vi "001_Calculate_DataSource.vi"(11 "Queue Ref In":T1={"UI"=refnum, "Message"=refnum, "Data"=refnum, "Caller"=refnum, "Name"="000 Common", "Data Path"=path "", "Class Path"=path "", "SubPanel"=refnum, "Project Name"="", "MNT"="", "Title"="", "Data Source"=refnum, "Queue List"={}, "VI"=refnum, "UE"=refnum}) -> ()   [LabVIEW 2020]
doc: "计算数据源"
uses:
  Alin/QMH/000 Module Data Type.ctl
  Alin/QMH/Queue Message.ctl
  <vilib>/Utility/miscctls.llb/LVRowAndColumnTypeDef.ctl
  <vilib>/Utility/file.llb/Read Delimited Spreadsheet (string).vi
  <vilib>/Utility/file.llb/Write Delimited Spreadsheet (string).vi
panel:
  in  "Formular List Refresh":bool
  in  "Formular Group Delete":bool
  in  "Formular Group Add":bool
  in  "Formular List":i32(listbox)
  in  "Warning Edit":bool
  in  "Formular Delete":bool
  in  "Formular Export":bool
  in  "Formular Import":bool
  in  "Formular Add":bool
  in  "Formular":i32(listbox)
  in  "Search":bool
  in  "Search Info":string
  in  "All Formular":i32(listbox)
  out "Delay":i32 format="Delay：%.0f ms"
  out "Numbers":i32 format="Sum：%.0f"
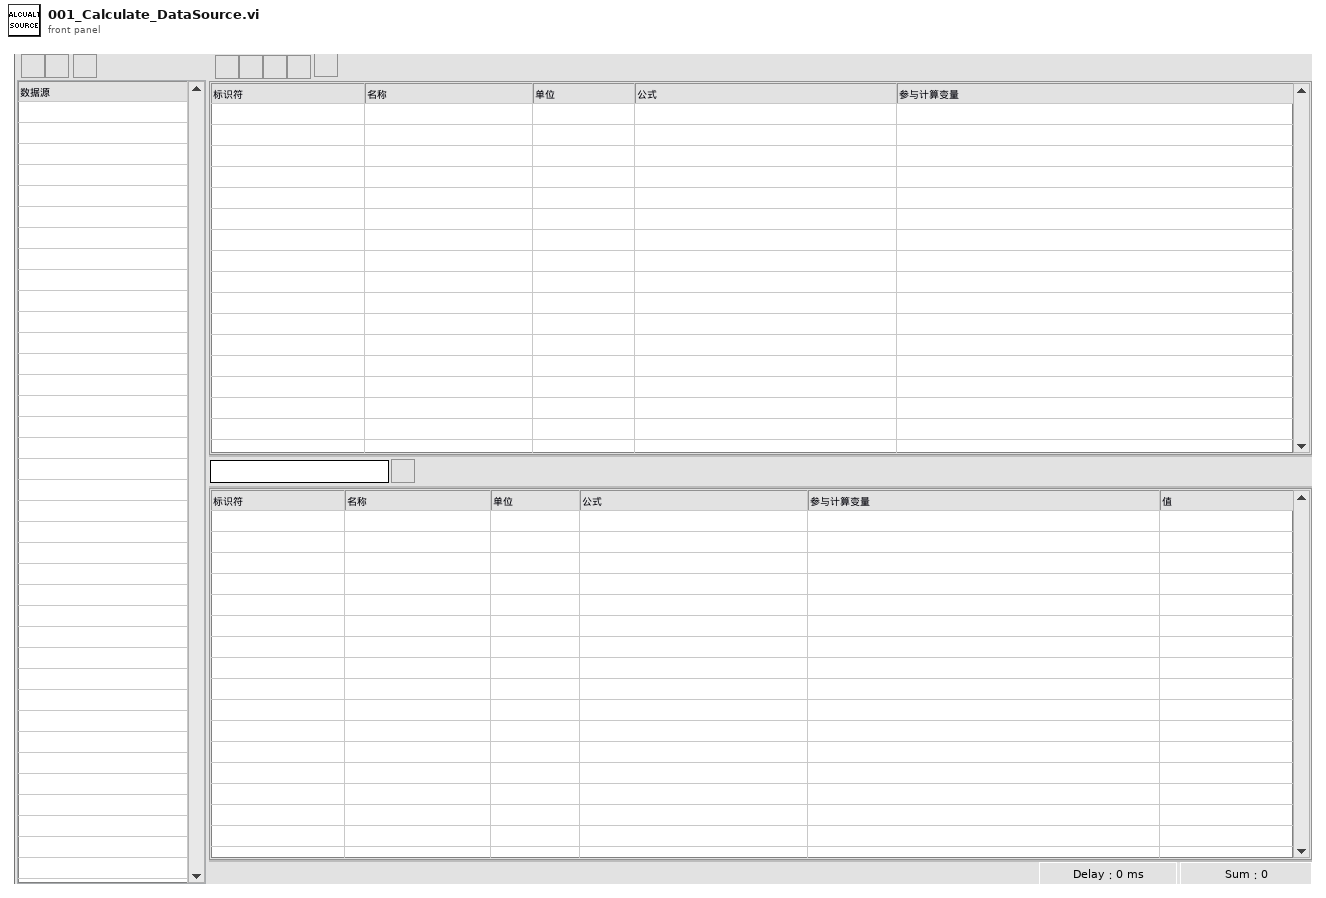
[diagram p1: front panel]
types:
  T1 = typedef "000 Module Data Type.ctl" = cluster{"UI":refnum<queue>, "Message":refnum<queue>, "Data":refnum<queue>, "Caller":refnum<queue>, "Name":string, "Data Path":path, "Class Path":path, "SubPanel":refnum<vi>, "Project Name":string, "MNT":string, "Title":string, "Data Source":refnum<queue>, "Queue List":map{string, refnum<queue>}, "VI":refnum<vi>, "UE":refnum<user-event>}
  T2 = cluster{"Queue":T1, "Formular":string[][], "Formular List":string[], "Last Time":u32, "Delay":u32, "Data Refresh":string}
  T3 = typedef "eventvkey.ctl" = enum16{"ASCII", "Enter", "Return", "Shift", "Ctrl", "Alt", "Cmd", "Opt", "Caps", "NumLock", "Clear", "Break", "Up", "Down", "Left", "Right", "Insert", "Delete", "Home", "End", "PageUp", "PageDown", "Escape", "Help", "Pause", "ScrollLock", "F1", "F2", "F3", "F4", "F5", "F6", "F7", "F8", "F9", "F10", "F11", "F12", "F13", "F14", "F15", "F16", "F17", "F18", "F19", "F20", "F21", "F22", "F23", "F24", "Play", "VolumeUp", "VolumeDown", "Mute", "Two Byte Char"}
  T4 = cluster{"Shift":bool, "Ctrl":bool, "Alt":bool, "Cmd":bool, "Opt":bool}
  T5 = typedef "LVPoint32TypeDef.ctl" = cluster{"Horizontal":i32, "Vertical":i32}
  T6 = typedef "LVRowAndColumnTypeDef.ctl" = cluster{"Row":i32, "Column":i32}
  T7 = cluster{"Formular":string[][], "Queue":T1, "FormularRef":refnum<vi>, "Formular ListRef":refnum<vi>, "Formular List":string[], "ForList Value":i32}
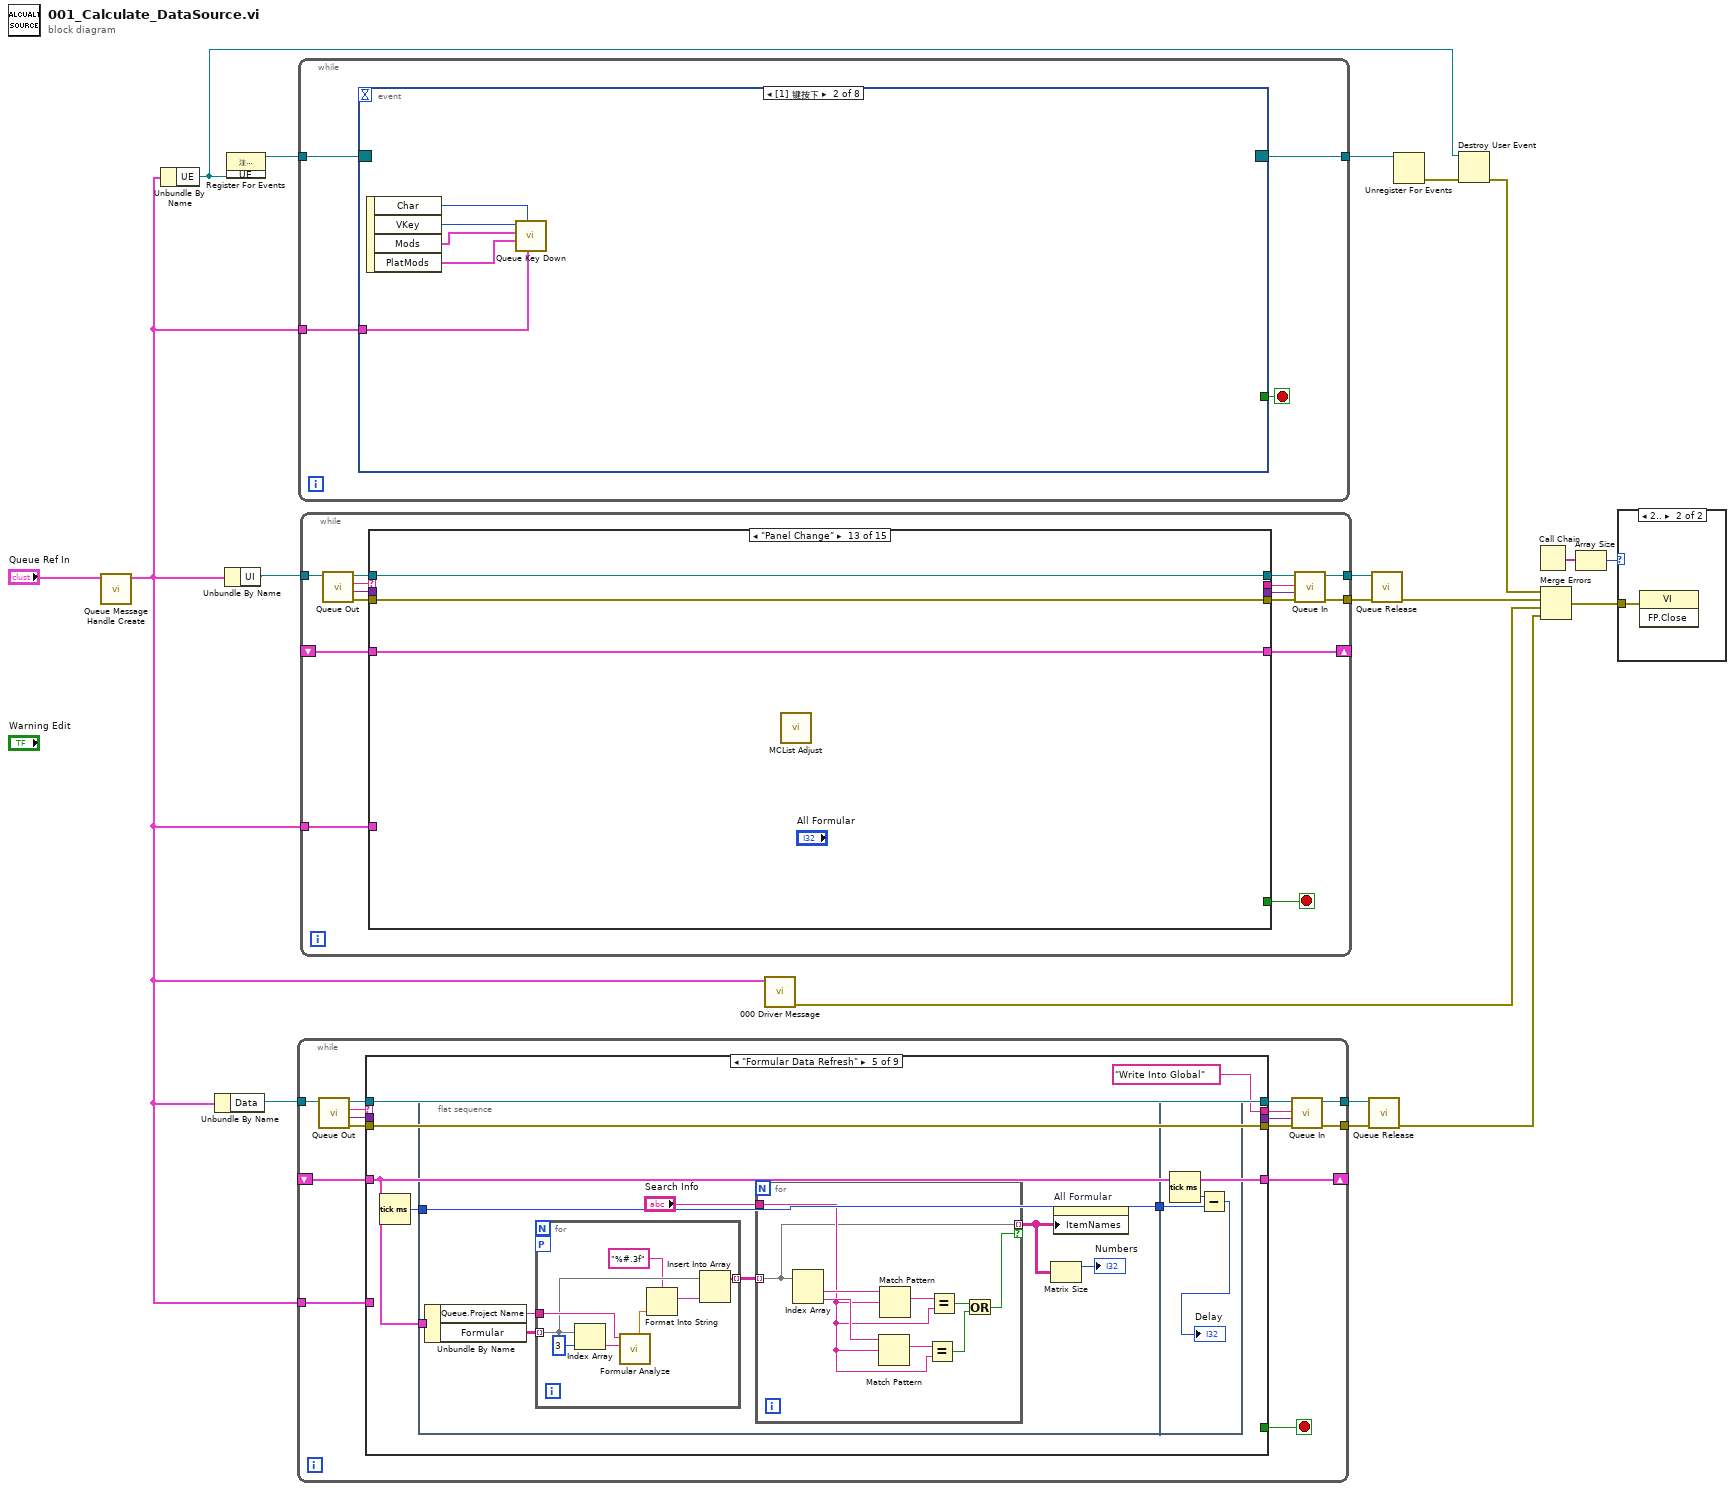
[diagram p0: block diagram]
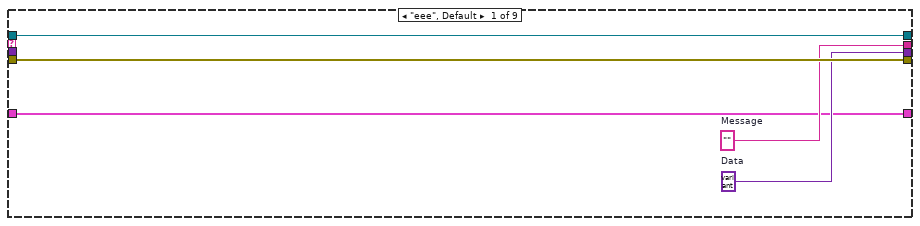
[diagram p2: hidden frame]
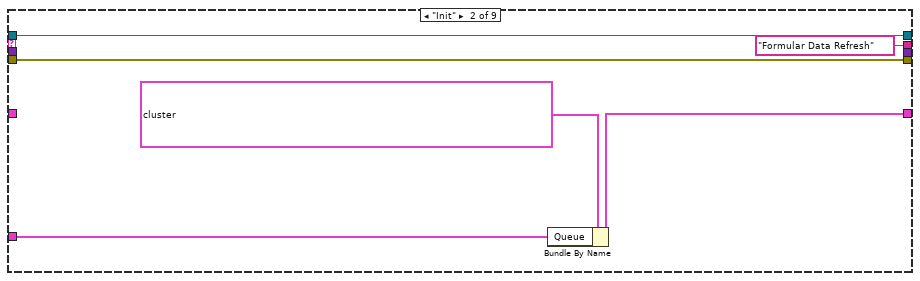
[diagram p3: hidden frame]
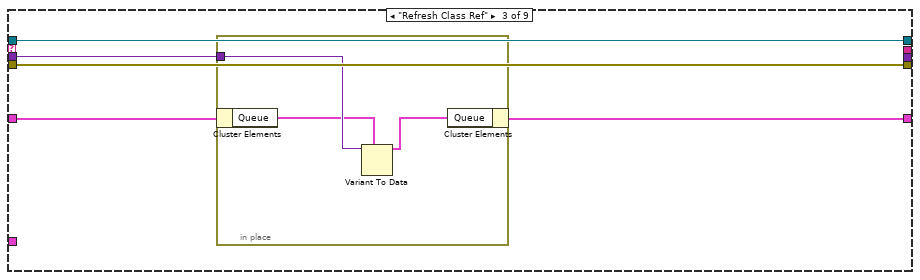
[diagram p4: hidden frame]
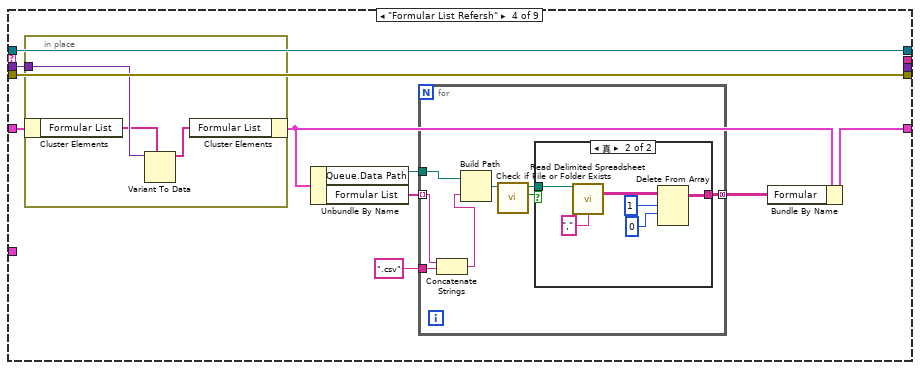
[diagram p5: hidden frame]
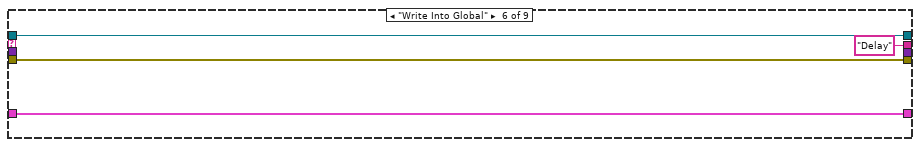
[diagram p7: hidden frame]
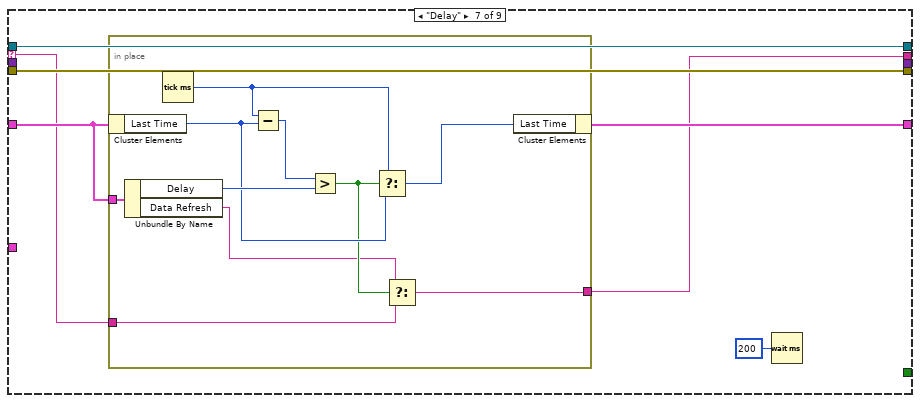
[diagram p8: hidden frame]
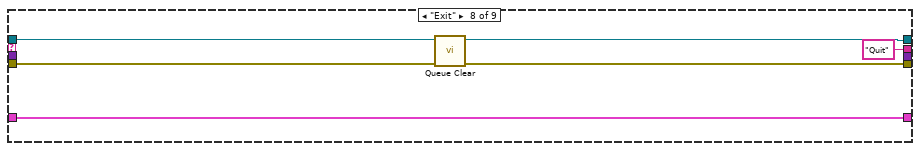
[diagram p9: hidden frame]
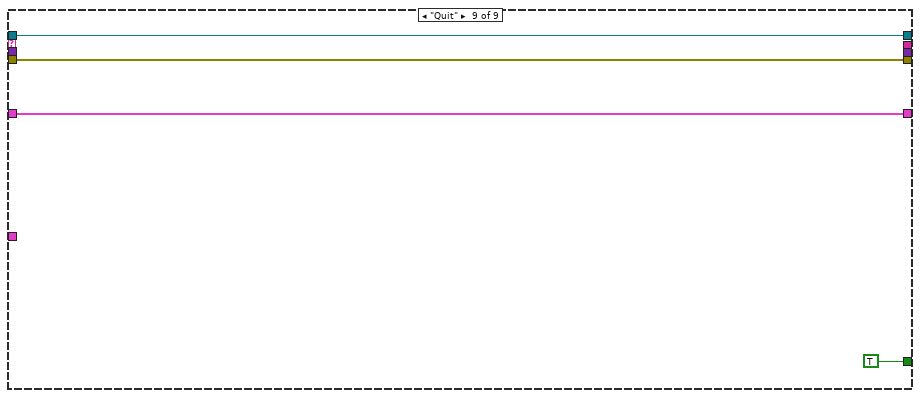
[diagram p10: hidden frame]
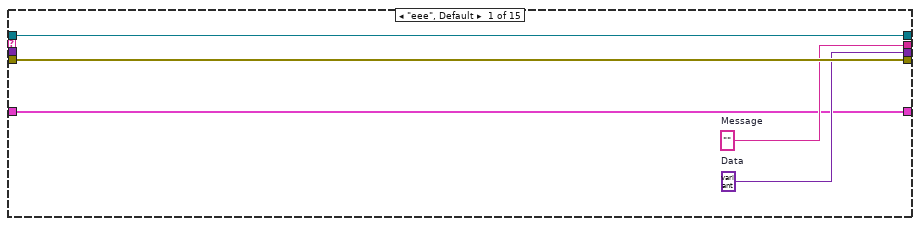
[diagram p12: hidden frame]
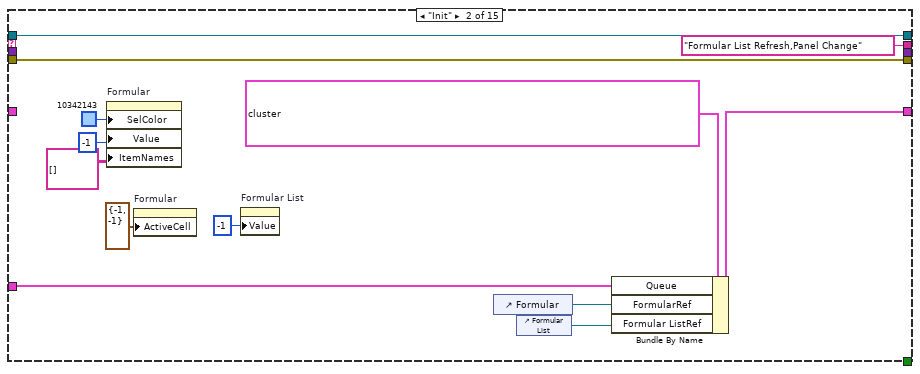
[diagram p13: hidden frame]
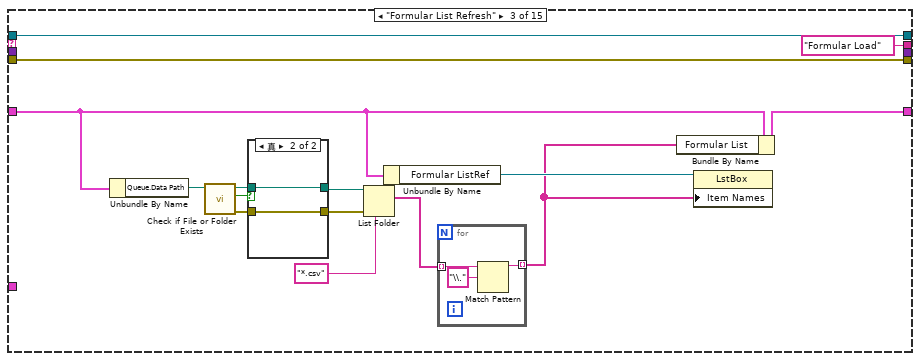
[diagram p14: hidden frame]
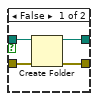
[diagram p15: hidden frame]
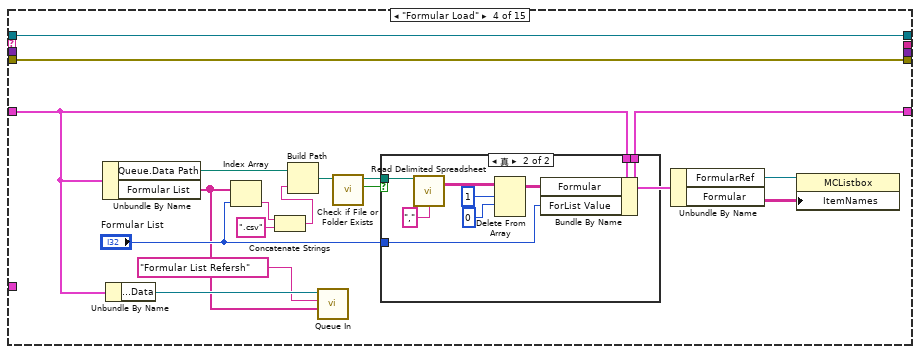
[diagram p16: hidden frame]
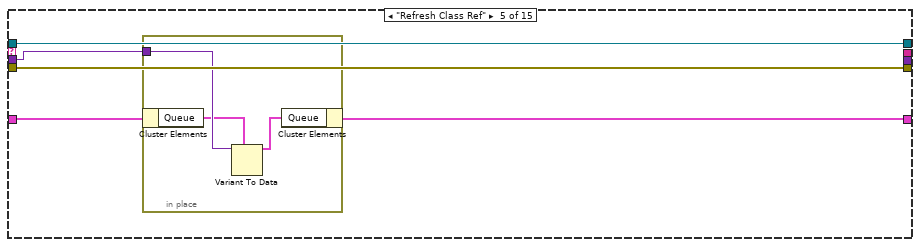
[diagram p18: hidden frame]
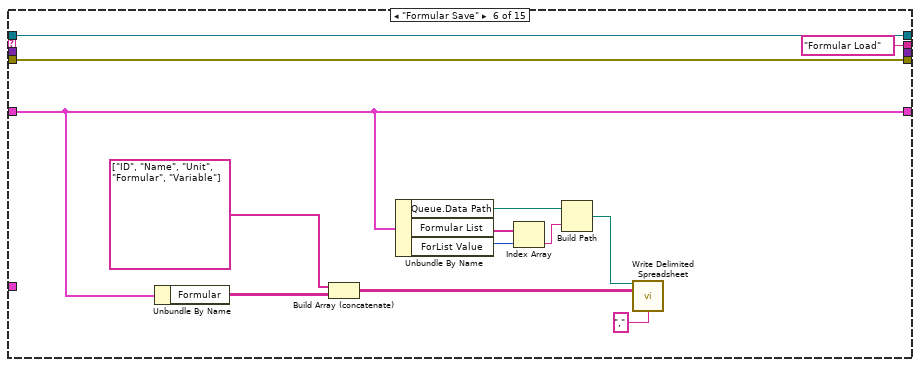
[diagram p19: hidden frame]
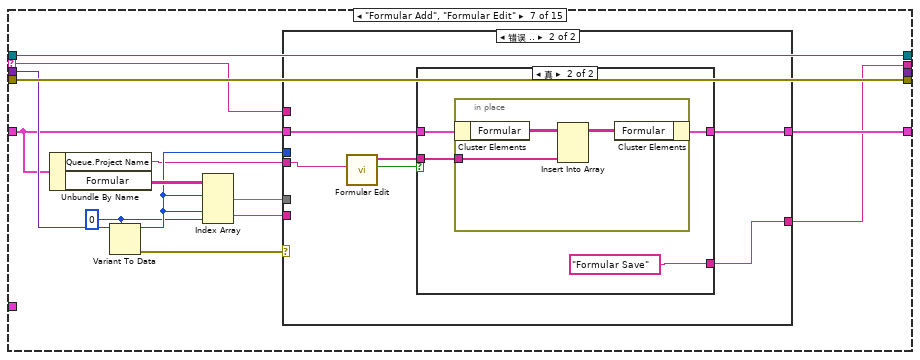
[diagram p20: hidden frame]
diagram:
  n1 = call "Queue Message Handle Create.vi"("Queue Ref In"="Queue Ref In") -> ("Queue Ref Out"=w1:T1)  [unwired: 9 in, 1 out]
  n2 = Unbundle By Name(w1) -> ("UE"=w2:refnum<user-event>)
  n3 = Unbundle By Name(w1) -> ("Data"=w17:refnum<queue>)
  n4 = Unbundle By Name(w1) -> ("UI"=w9:refnum<queue>)
  n5 = register-events(w2) -> (reference out=w4:refnum<event-registration>)  [unwired: 2 in, 1 out]
  n6 = while {
    tunnel: w17 -> [w30]
    tunnel: [w27] -> w15
    tunnel: [w26] -> w16
    shift-right: [w22] -> _
    shift-left: _ -> [w21]
    tunnel: w1 -> [w20]
    stop <- w34 stop-if-true
    n7 = call "Queue Out.vi"("Queue In"=w30) -> ("error out"=w33:errorcluster, "Data"=w31:variant, "Message"=w32:string, "Queue Out"=w29:refnum<queue>)  [unwired: 6 in, 1 out]
    n8 = case shown="\"Formular Data Refresh\"" w32 {
      selector: w32 -> [_ _ _ _ _ _ w120 _ _]
      tunnel: w29 -> [w39 w45 w50 w63 w86 w118 w125 w140 w144]
      tunnel: w33 -> [w38 w44 w49 w62 w85 w117 w124 w138 w145]
      tunnel: [w39 w45 w50 w63 w86 w118 w125 w139 w144] -> w28
      tunnel: [w38 w44 w49 w62 w85 w117 w124 w137 w145] -> w25
      tunnel: [w37 "Formular Data Refresh" ("Message") _ _ "Write Into Global" ("Message") "Delay" ("Data Refresh") w119 "Quit" _] -> w24
      tunnel: [_ _ _ _ _ _ _ _ TRUE] -> w34
      tunnel: [w36 _ _ _ _ _ _ _ _] -> w23
      tunnel: w31 -> [_ _ w46 w60 _ _ _ _ _]
      tunnel: [w35 w42 w47 w56 w83 w116 w122 w136 w142] -> w22
      tunnel: w21 -> [w35 _ w48 w61 w83 w116 w121 w136 w142]
      tunnel: w20 -> [_ w41 _ _ _ _ _ _ _]
      frame "eee", Default {
        w36 = variant  # Data
        w37 = ""  # Message
      }
      frame "Init" {
        n9 = Bundle By Name(cluster=T2 {"Queue"={"UI"=refnum, "Message"=refnum, "Data"=refnum, "Caller"=refnum, "Name"="000 Common", "Data Path"=path "", "Class Path"=path "", "SubPanel"=refnum, "Project Name"="", "MNT"="", "Title"="", "Data Source"=refnum, "Queue List"={}, "VI"=refnum, "UE"=refnum}, "Formular"=[], "Formular List"=[], "Last Time"=0, "Delay"=500, "Data Refresh"="Formular Data Refresh"}, "Queue"=w41) -> (w42:T2)
      }
      frame "Refresh Class Ref" {
        n10 = in-place {
          in-place-border: w46 -> [w53]
          n11 = in-place-cluster #1(w48) -> ("Queue"=w52:T1)
          n12 = Variant To Data(type=w52, Variant=w53) -> (data=w51:T1)  [unwired: 1 in, 1 out]
          n13 = in-place-cluster #1("Queue"=w51) -> (w47:T2)
        }
      }
      frame "Formular List Refersh" {
        n14 = in-place {
          in-place-border: w60 -> [w80]
          n15 = in-place-cluster #2(w61) -> ("Formular List"=w79:string[])
          n16 = Variant To Data(type=w79, Variant=w80) -> (data=w78:string[])  [unwired: 1 in, 1 out]
          n17 = in-place-cluster #2("Formular List"=w78) -> (w59:T2)
        }
        n18 = Unbundle By Name(w59) -> ("Queue.Data Path"=w58:path, "Formular List"=w57:string[])
        n19 = for {
          tunnel: w58 -> [w70]
          tunnel: w57 -> [w65] mode=indexing
          tunnel: [w67] -> w55 mode=concatenating
          tunnel: ".csv" ("字符串") -> [w66]
          n20 = Concatenate Strings(w65, w66) -> (w64:string)
          n21 = Build Path(base path=w70, name or relative path=w64) -> (appended path=w71:path)
          n22 = call <vilib>:"Check if File or Folder Exists.vi"("path"=w71) -> ("file or folder exists?"=w69:bool, "dup path"=w68:path)  [unwired: 8 in, 1 out]
          n23 = case shown="真" w69 {
            tunnel: w68 -> [_ w74]
            tunnel: [_ w72] -> w67
            frame False {
            }
            frame True {
              n24 = call-poly <vilib>:"Read Delimited Spreadsheet.vi"("file path (dialog if empty)"=w74, "delimiter (\\t)"="," ("delimiter (\\t)")) -> ("all rows"=w73:string[][])  [unwired: 8 in, 5 out]
              n25 = Delete From Array(array=w73, length=1 ("长度"), index (row)=0 ("索引 (行)")) -> (array with subset deleted=w72:string[][])  [unwired: 1 in, 1 out]
            }
          }
        }
        n26 = Bundle By Name(cluster=w59, "Formular"=w55) -> (w56:T2)
      }
      frame "Formular Data Refresh" {
        n27 = Tick Count (ms)() -> (millisecond timer value=w82:u32)
        n28 = flat-sequence {
          tunnel: w83 -> [w94]
          tunnel: w82 -> [w87]
          tunnel: [w87] -> w81
          tunnel: w81 -> [w113]
          frame #0 {
            n29 = Unbundle By Name(w94) -> ("Queue.Project Name"=w92:string, "Formular"=w93:string[][])
            n30 = for {
              workers-P: _ -> [_]
              tunnel: w93 -> [w108] mode=indexing
              tunnel: w92 -> [w109]
              tunnel: [w107] -> w91 mode=indexing
              n31 = Index Array(array=w108, index=3 ("索引")) -> (element=w110:string)
              n32 = call "Formular Analyze.vi"("Formular"=w110, "Project"=w109) -> ("Value"=w105:dbl)  [unwired: 5 in, 4 out]
              n33 = Format Into String(format string="%#.3f" ("格式字符串"), w105) -> (resulting string=w104:string)  [unwired: 2 in, 1 out]
              n34 = Insert Into Array(array=w108, new element=w104) -> (w107:string[])  [unwired: 1 in]
            }
            n35 = for {
              tunnel: w91 -> [w97] mode=indexing
              tunnel: "Search Info" -> [w100]
              tunnel: [w97] -> w89 mode=indexing if=w96
              n36 = Index Array(array=w97) -> (element #1=w103:string, element #2=w102:string)  [unwired: 2 in]
              n37 = Match Pattern(string=w102, regular expression=w100) -> (match substring=w95:string)  [unwired: 1 in, 3 out]
              n38 = Match Pattern(string=w103, regular expression=w100) -> (match substring=w101:string)  [unwired: 1 in, 3 out]
              n39 = Equal?(x=w95, y=w100) -> (x = y?=w98:bool)
              n40 = Equal?(x=w101, y=w100) -> (x = y?=w99:bool)
              n41 = Or(x=w99, y=w98) -> (x .or. y?=w96:bool)
            }
            n42 = Matrix Size(0:w89) -> (1:→"Numbers":i32)  [unwired: 1 out]
            n43 = property on="All Formular" class="MCListbox (严格)"("ItemNames"=w89) -> ()  [unwired: 2 in, 2 out]
          }
          frame #1 {
            n44 = Tick Count (ms)() -> (millisecond timer value=w114:u32)
            n45 = Subtract(x=w114, y=w113) -> (x-y=→"Delay":u32)
          }
        }
      }
      frame "Write Into Global" {
      }
      frame "Delay" {
        n46 = in-place {
          in-place-border: w121 -> [w134]
          in-place-border: w120 -> [w128]
          in-place-border: [w127] -> w119
          n47 = in-place-cluster #3(w121) -> ("Last Time"=w130:u32)
          n48 = Unbundle By Name(w134) -> ("Delay"=w133:u32, "Data Refresh"=w126:string)
          n49 = Tick Count (ms)() -> (millisecond timer value=w132:u32)
          n50 = Subtract(x=w132, y=w130) -> (x-y=w135:u32)
          n51 = Greater?(x=w135, y=w133) -> (0:w129:bool)
          n52 = Select(t=w132, s=w129, f=w130) -> (s? t:f=w131:u32)
          n53 = Select(t=w126, s=w129, f=w128) -> (s? t:f=w127:string)
          n54 = in-place-cluster #3("Last Time"=w131) -> (w122:T2)
        }
        n55 = Wait (ms)(milliseconds to wait=u32 200 ("等待时间（毫秒）")) -> ()  [unwired: 1 out]
      }
      frame "Exit" {
        n56 = call "Queue Clear.vi"("error in (no error)"=w138, "Queue In"=w140) -> ("error out"=w137:errorcluster, "Queue Out"=w139:refnum<queue>)  [unwired: 8 in]
      }
      frame "Quit" {
      }
    }
    n57 = call "Queue In.vi"("error in (no error)"=w25, "Data"=w23, "Message"=w24, "Queue In"=w28) -> ("error out"=w26:errorcluster, "Queue Out"=w27:refnum<queue>)  [unwired: 6 in]
  }
  n58 = while {
    tunnel: w4 -> [w149]
    tunnel: [w147] -> w5
    tunnel: w1 -> [w146]
    stop <- w148 stop-if-true
    n59 = event shown="[1] 键按下" {
      selector: w149 -> [_ _ _ _ _ _ _ _]
      dyn-events: [_ _ _ _ _ _ _ _] -> w147
      timeout: _ -> [_ _ _ _ _ _ _ _]
      tunnel: [_ _ _ w158 _ _ _ _] -> w148
      tunnel: w146 -> [_ w150 w157 _ w163 w179 w185 w189]
      event Timeout {
        n60 = event-data() -> ()  [unwired: 1 in, 1 out]
      }
      event Key Down {
        n61 = event-data() -> ("Char"=w154:i16, "VKey"=w153:T3, "Mods"=w152:cluster{"Num Pad":bool, "Menu Key":bool}, "PlatMods"=w151:T4)  [unwired: 1 in]
        n62 = call "Queue Key Down.vi"("Queue Ref Out"=w150, "C"=w154, "Platform Key"=w151, "Group Key"=w152, "V Key"=w153) -> ()  [unwired: 6 in, 1 out]
      }
      event Panel Resize {
        n63 = event-data() -> ()  [unwired: 1 in, 1 out]
        n64 = Unbundle By Name(w157) -> ("Message"=w156:refnum<queue>)
        n65 = call "Queue In.vi"("Message"="Panel Change", "Queue In"=w156) -> ()  [unwired: 8 in, 2 out]
      }
      event User Event {
        n66 = event-data() -> ("Message"=w160:string)  [unwired: 1 in]
        n67 = Equal?(x=w160, y="Exit") -> (x = y?=w158:bool)
      }
      event Panel Close? {
        n68 = event-data() -> ()  [unwired: 1 in, 1 out]
        n69 = Call Chain() -> (call chain=w165:string[])
        n70 = Array Size(array=w165) -> (size(s)=w164:i32)
        n71 = case shown="1" w164 {
          tunnel: w163 -> [w169 w172]
          tunnel: [w168 w171] -> w162
          tunnel: ["Panel Hidden" ("Message") "Exit Prepare" ("Message")] -> w161
          frame 2, Default {
            n72 = Unbundle By Name(w169) -> ("Message"=w168:refnum<queue>)
          }
          frame 1 {
            n73 = Unbundle By Name(w172) -> ("Message"=w171:refnum<queue>)
          }
        }
        n74 = call "Queue In.vi"("Message"=w161, "Queue In"=w162) -> ()  [unwired: 8 in, 2 out]
        n75 = event-data("Discard?"=TRUE ("放弃？")) -> ()  [unwired: 1 in, 1 out]
      }
      event "Formular": Double Click {
        n76 = event-data() -> ("CtlRef"=w177:refnum<vi>, "Coords"=w176:T5)  [unwired: 1 in]
        n77 = Unbundle By Name(w179) -> ("UI"=w178:refnum<queue>)
        n78 = invoke class="MCListbox (严格)" method="Point To Row Column"(reference=w177, "Point"=w176) -> ("CellPosition"=w175:T6)  [unwired: 5 in, 6 out]
        n79 = Unbundle By Name(w175) -> ("Column"=w174:i32, "Row"=w173:i32)
        n80 = case shown="3" w174 {
          tunnel: w178 -> [_ w182]
          tunnel: w173 -> [_ w180]
          frame 0, Default {
          }
          frame 3 {
            n81 = call "Queue In.vi"("Data"=w180, "Message"="Formular Edit", "Queue In"=w182) -> ()  [unwired: 7 in, 2 out]
          }
        }
      }
      event "Formular Add", "Formular Group Add", "Formular Group Delete", "Formular Import", "Formular Export", "Formular Delete", "Formular List Refresh": Value Change {
        n82 = event-data() -> ("CtlRef"=w186:refnum<vi>)  [unwired: 1 in]
        n83 = property class="Bool"(reference=w186) -> ("Label.Text"=w183:string)  [unwired: 1 in, 2 out]
        n84 = Unbundle By Name(w185) -> ("UI"=w184:refnum<queue>)
        n85 = call "Queue In.vi"("Message"=w183, "Queue In"=w184) -> ()  [unwired: 8 in, 2 out]
      }
      event "Formular List": Value Change {
        n86 = event-data() -> ()  [unwired: 1 in, 1 out]
        n87 = Unbundle By Name(w189) -> ("UI"=w188:refnum<queue>)
        n88 = call "Queue In.vi"("Message"="Formular Load", "Queue In"=w188) -> ()  [unwired: 8 in, 2 out]
      }
    }
  }
  n89 = while {
    tunnel: w9 -> [w200]
    tunnel: [w197] -> w7
    tunnel: [w196] -> w8
    tunnel: w1 -> [w192]
    shift-right: [w191] -> _
    shift-left: _ -> [w190]
    stop <- w204 stop-if-true
    n90 = call "Queue Out.vi"("Queue In"=w200) -> ("error out"=w203:errorcluster, "Data"=w201:variant, "Message"=w202:string, "Queue Out"=w199:refnum<queue>)  [unwired: 6 in, 1 out]
    n91 = case shown="\"Panel Change\"" w202 {
      selector: w202 -> [_ _ _ _ _ _ w298 _ _ _ _ _ _ w451 _]
      tunnel: w199 -> [w209 w222 w237 w263 w278 w294 w308 w359 w381 w391 w413 w437 w448 w458 w464]
      tunnel: w203 -> [w208 w221 w236 w262 w277 w293 w307 w358 w380 w390 w412 w436 w447 w456 w465]
      tunnel: [w209 w222 w237 w263 w278 w294 w308 w359 w381 w391 w413 w437 w448 w457 w464] -> w198
      tunnel: [w208 w221 w236 w262 w277 w293 w307 w358 w380 w390 w412 w436 w447 w455 w465] -> w195
      tunnel: [w207 "Formular List Refresh,Panel Change" ("Message") "Formular Load" ("Message") _ _ "Formular Load" ("Message") w301 "Formular List Refresh" ("Message") "Formular List Refresh" ("Message") _ w404 w433 _ "Quit" _] -> w194
      tunnel: [_ _ _ _ _ _ _ _ _ _ _ _ _ _ TRUE] -> w204
      tunnel: [w206 _ _ _ _ _ _ _ _ _ _ _ _ _ _] -> w193
      tunnel: w201 -> [_ _ _ _ w274 _ w306 _ _ _ _ _ _ _ _]
      tunnel: w192 -> [_ w210 _ _ _ _ _ _ _ _ _ _ _ _ _]
      tunnel: [w205 w218 w226 w258 w275 w290 w302 w355 w379 w384 w406 w435 w446 w449 w462] -> w191
      tunnel: w190 -> [w205 _ w229 w253 w276 w290 w305 w355 w379 w385 w407 w434 w446 w449 w462]
      frame "eee", Default {
        w206 = variant  # Data
        w207 = ""  # Message
      }
      frame "Init" {
        n92 = property on="Formular" class="MCListbox (严格)"("SelColor"=u32 10342143 ("选择颜色"), "Value"=-1 ("Formular"), "ItemNames"=string[][] [] ("项名")) -> ()  [unwired: 2 in, 2 out]
        n93 = property on="Formular" class="MCListbox (严格)"("ActiveCell"=T6 {"Row"=-1, "Column"=-1} ("活动单元格:活动单元格")) -> ()  [unwired: 2 in, 2 out]
        n94 = property on="Formular List" class="LstBox (严格)"("Value"=-1 ("Formular List")) -> ()  [unwired: 2 in, 2 out]
        n95 = control-ref of="Formular"() -> (w216:refnum<vi>)
        n96 = control-ref of="Formular List"() -> (w215:refnum<vi>)
        n97 = Bundle By Name(cluster=T7 {"Formular"=[], "Queue"={"UI"=refnum, "Message"=refnum, "Data"=refnum, "Caller"=refnum, "Name"="000 Common", "Data Path"=path "", "Class Path"=path "", "SubPanel"=refnum, "Project Name"="", "MNT"="", "Title"="", "Data Source"=refnum, "Queue List"={}, "VI"=refnum, "UE"=refnum}, "FormularRef"=refnum, "Formular ListRef"=refnum, "Formular List"=[], "ForList Value"=0}, "Queue"=w210, "FormularRef"=w216, "Formular ListRef"=w215) -> (w218:T7)
      }
      frame "Formular List Refresh" {
        n98 = Unbundle By Name(w229) -> ("Queue.Data Path"=w235:path)
        n99 = call <vilib>:"Check if File or Folder Exists.vi"("path"=w235) -> ("error out"=w232:errorcluster, "file or folder exists?"=w234:bool, "dup path"=w233:path)  [unwired: 8 in]
        n100 = case shown="真" w234 {
          tunnel: w233 -> [w244 w246]
          tunnel: w232 -> [w243 w245]
          tunnel: [w241 w246] -> w231
          tunnel: [w242 w245] -> w230
          frame False {
            n101 = Create Folder(path (use dialog)=w244, error in=w243) -> (created path=w241:path, error out=w242:errorcluster)  [unwired: 1 in, 1 out]
          }
          frame True {
          }
        }
        n102 = List Folder(path=w231, pattern="*.csv" ("类型"), error in=w230) -> (filenames=w224:string[])  [unwired: 1 in, 3 out]
        n103 = Unbundle By Name(w229) -> ("Formular ListRef"=w228:refnum<vi>)
        n104 = for {
          tunnel: w224 -> [w240] mode=indexing
          tunnel: [w238] -> w223 mode=indexing
          n105 = Match Pattern(string=w240, regular expression="\\." ("正则表达式")) -> (before substring=w238:string)  [unwired: 1 in, 3 out]
        }
        n106 = Bundle By Name(cluster=w229, "Formular List"=w223) -> (w226:T7)
        n107 = property class="LstBox"(reference=w228, "Item Names"=w223) -> ()  [unwired: 1 in, 2 out]
      }
      frame "Formular Load" {
        n108 = Unbundle By Name(w253) -> ("Queue.Data Path"=w261:path, "Formular List"=w251:string[])
        n109 = Unbundle By Name(w253) -> ("Queue.Data"=w252:refnum<queue>)
        n110 = Index Array(array=w251, index="Formular List") -> (element=w249:string)
        n111 = Concatenate Strings(w249, ".csv" ("字符串")) -> (w247:string)
        n112 = Build Path(base path=w261, name or relative path=w247) -> (appended path=w256:path)
        n113 = call "Queue In.vi"("Data"=w251, "Message"="Formular List Refersh", "Queue In"=w252) -> ()  [unwired: 7 in, 2 out]
        n114 = call <vilib>:"Check if File or Folder Exists.vi"("path"=w256) -> ("file or folder exists?"=w255:bool, "dup path"=w254:path)  [unwired: 8 in, 1 out]
        n115 = case shown="真" w255 {
          tunnel: w253 -> [w264 w273]
          tunnel: [w264 w267] -> w258
          tunnel: "Formular List" -> [_ w266]
          tunnel: w254 -> [_ w265]
          frame False {
          }
          frame True {
            n116 = call-poly <vilib>:"Read Delimited Spreadsheet.vi"("file path (dialog if empty)"=w265, "delimiter (\\t)"="," ("delimiter (\\t)")) -> ("all rows"=w268:string[][])  [unwired: 8 in, 5 out]
            n117 = Delete From Array(array=w268, length=1 ("长度"), index (row)=0 ("索引 (行)")) -> (array with subset deleted=w271:string[][])  [unwired: 1 in, 1 out]
            n118 = Bundle By Name(cluster=w273, "Formular"=w271, "ForList Value"=w266) -> (w267:T7)
          }
        }
        n119 = Unbundle By Name(w258) -> ("FormularRef"=w259:refnum<vi>, "Formular"=w260:string[][])
        n120 = property on="属性节点" class="MCListbox"(reference=w259, "ItemNames"=w260) -> ()  [unwired: 1 in, 2 out]
      }
      frame "Refresh Class Ref" {
        n121 = in-place {
          in-place-border: w274 -> [w281]
          n122 = in-place-cluster #4(w276) -> ("Queue"=w280:T1)
          n123 = Variant To Data(type=w280, Variant=w281) -> (data=w279:T1)  [unwired: 1 in, 1 out]
          n124 = in-place-cluster #4("Queue"=w279) -> (w275:T7)
        }
      }
      frame "Formular Save" {
        n125 = Unbundle By Name(w290) -> ("Formular"=w291:string[][])
        n126 = Build Array (concatenate)(string[] ["ID", "Name", "Unit", "Formular", "Variable"], w291) -> (w287:string[][])
        n127 = Unbundle By Name(w290) -> ("Queue.Data Path"=w286:path, "Formular List"=w285:string[], "ForList Value"=w284:i32)
        n128 = Index Array(array=w285, index=w284) -> (element=w283:string)
        n129 = Build Path(base path=w286, name or relative path=w283) -> (appended path=w282:path)
        n130 = call-poly <vilib>:"Write Delimited Spreadsheet.vi"("file path (dialog if empty)"=w282, "2D data"=w287, "delimiter (\\t)"="," ("delimiter (\\t)")) -> ()  [unwired: 11 in, 2 out]
      }
      frame "Formular Add", "Formular Edit" {
        w299 = 0 ("Row")
        n131 = Unbundle By Name(w305) -> ("Queue.Project Name"=w295:string, "Formular"=w304:string[][])
        n132 = Variant To Data(type=w299, Variant=w306) -> (data=w300:i32, error out=w297:errorcluster)  [unwired: 1 in]
        n133 = Index Array(array=w304, index (row) #1=w300, index (row) #2=w300, index (col) #2=w299) -> (element #1=w303:string[], element #2=w296:string)  [unwired: 1 in]
        n134 = case shown="错误 .." w297 {
          tunnel: w305 -> [w316 w344]
          tunnel: w303 -> [w315 _]
          tunnel: [w314 w342] -> w302
          tunnel: w300 -> [w313 _]
          tunnel: [w312 w341] -> w301
          tunnel: w298 -> [w311 _]
          tunnel: w296 -> [w310 _]
          tunnel: w295 -> [w309 w340]
          frame No Error {
            n135 = case shown="\"eee\", 默认" w310 {
              tunnel: w316 -> [w325 w339]
              tunnel: w315 -> [w324 _]
              tunnel: [w323 w339] -> w314
              tunnel: w313 -> [w321 _]
              tunnel: [w319 _] -> w312
              tunnel: w311 -> [w318 _]
              tunnel: w309 -> [w317 _]
              frame "eee", Default {
                n136 = call "Formular Edit.vi"("Project"=w317, "Identifier In"=w324) -> ("OK?"=w320:bool, "Identifier In"=w322:string[])  [unwired: 8 in]
                n137 = in-place {
                  in-place-border: w322 -> [w330]
                  in-place-border: w321 -> [w329]
                  in-place-border: w320 -> [w328]
                  in-place-border: [w327] -> w319
                  in-place-border: w318 -> [w326]
                  n138 = in-place-cluster #5(w325) -> ("Formular"=w332:string[][])
                  n139 = case shown="真" w328 {
                    tunnel: w332 -> [w333 w338]
                    tunnel: [w333 w337] -> w331
                    tunnel: w330 -> [_ w336]
                    tunnel: w329 -> [_ w335]
                    tunnel: [_ "Formular Save"] -> w327
                    tunnel: w326 -> [_ _]
                    frame False {
                    }
                    frame True {
                      n140 = Replace Array Subset(array=w338, new element=w336, index (row)=w335) -> (w337:string[][])  [unwired: 1 in]
                    }
                  }
                  n141 = in-place-cluster #5("Formular"=w331) -> (w323:T7)
                }
              }
              frame "" {
              }
            }
          }
          frame Error {
            n142 = call "Formular Edit.vi"("Project"=w340) -> ("OK?"=w345:bool, "Identifier In"=w343:string[])  [unwired: 9 in]
            n143 = case shown="真" w345 {
              tunnel: w344 -> [w346 w350]
              tunnel: w343 -> [_ w347]
              tunnel: [w346 w348] -> w342
              tunnel: [_ "Formular Save"] -> w341
              frame False {
              }
              frame True {
                n144 = in-place {
                  in-place-border: w347 -> [w352]
                  n145 = in-place-cluster #6(w350) -> ("Formular"=w353:string[][])
                  n146 = Insert Into Array(array=w353, new element=w352) -> (w351:string[][])  [unwired: 2 in]
                  n147 = in-place-cluster #6("Formular"=w351) -> (w348:T7)
                }
              }
            }
          }
        }
      }
      frame "Formular Group Add" {
        n148 = call "Data Source Add Group.vi"() -> ("OK？"=w356:bool, "Data Out"=w357:string[])  [unwired: 9 in, 1 out]
        n149 = case shown="真" w356 {
          tunnel: w357 -> [_ w369]
          tunnel: w355 -> [_ w368]
          frame False {
          }
          frame True {
            n150 = Unbundle By Name(w368) -> ("Queue.Data Path"=w367:path)
            n151 = Index Array(array=w369) -> (element=w365:string)  [unwired: 1 in]
            n152 = Format Into String(format string="%s.csv" ("格式字符串"), w365) -> (resulting string=w364:string)  [unwired: 2 in, 1 out]
            n153 = Build Path(base path=w367, name or relative path=w364) -> (appended path=w363:path)
            n154 = call-poly <vilib>:"Write Delimited Spreadsheet.vi"("file path (dialog if empty)"=w363, "2D data"=string[][] [], "append to file? (new file:F)"=TRUE, "delimiter (\\t)"="," ("delimiter (\\t)")) -> ()  [unwired: 10 in, 2 out]
          }
        }
      }
      frame "Formular Group Delete" {
        n155 = Unbundle By Name(w379) -> ("Queue.Data Path"=w378:path, "Formular List"=w377:string[], "ForList Value"=w376:i32)
        n156 = Index Array(array=w377, index=w376) -> (element=w375:string)
        n157 = Build Path(base path=w378, name or relative path=w375) -> (appended path=w374:path)
        n158 = call <vilib>:"Check if File or Folder Exists.vi"("path"=w374) -> ("error out"=w371:errorcluster, "file or folder exists?"=w373:bool, "dup path"=w372:path)  [unwired: 8 in]
        n159 = case shown="真" w373 {
          tunnel: w372 -> [_ w383]
          tunnel: w371 -> [_ w382]
          frame False {
          }
          frame True {
            n160 = Delete(path (use dialog)=w383, error in=w382) -> ()  [unwired: 3 in, 3 out]
          }
        }
      }
      frame "Formular Export" {
        n161 = call "文件对话框"("pattern (all files)"="*.xlsx") -> ("selected path"=w388:path, "cancelled"=w386:bool, "error out"=w387:errorcluster)  [unwired: 11 in, 1 out]
        n162 = case shown="无错误" w387 {
          tunnel: w388 -> [w392 _]
          tunnel: w386 -> [w395 _]
          tunnel: w385 -> [w394 w403]
          tunnel: [w393 w403] -> w384
          frame No Error {
            n163 = case shown="假" w395 {
              tunnel: w394 -> [w401 w402]
              tunnel: [w401 w402] -> w393
              tunnel: w392 -> [w400 _]
              frame False {
                n164 = Unbundle By Name(w401) -> ("FormularRef"=w399:refnum<vi>, "Formular"=w397:string[][])
                n165 = property class="MCListbox"(reference=w399) -> ("ColHdrString"=w398:string[])  [unwired: 1 in, 2 out]
                n166 = Build Array (concatenate)(w398, w397) -> (w396:string[][])
                n167 = call "Excel Write.vi"("Write"=w396, "Path"=w400) -> ()  [unwired: 9 in, 1 out]
              }
              frame True {
              }
            }
          }
          frame Error {
          }
        }
      }
      frame "Formular Import" {
        n168 = call "文件对话框2"("pattern (all files)"="*.xlsx") -> ("selected path"=w405:path, "exists"=w408:bool, "cancelled"=w409:bool, "error out"=w410:errorcluster)  [unwired: 11 in]
        n169 = case shown="无错误" w410 {
          tunnel: w409 -> [_ _]
          tunnel: w408 -> [w418 _]
          tunnel: w407 -> [w417 w432]
          tunnel: [w416 w432] -> w406
          tunnel: w405 -> [w415 _]
          tunnel: [w414 _] -> w404
          frame No Error {
            n170 = case shown="真" w418 {
              tunnel: w417 -> [w419 w423]
              tunnel: [w419 w422] -> w416
              tunnel: w415 -> [_ w421]
              tunnel: [_ w420] -> w414
              frame False {
              }
              frame True {
                n171 = in-place {
                  in-place-border: w421 -> [w431]
                  in-place-border: ["Formular Save"] -> w420
                  n172 = in-place-cluster #7(w423) -> ("Formular"=w427:string[][])
                  n173 = call "Excel Read.vi"("Path"=w431) -> ("Read"=w430:string[][])  [unwired: 9 in, 1 out]
                  n174 = Delete From Array(array=w430, length=1 ("长度"), index (row)=0 ("索引 (行)")) -> (array with subset deleted=w425:string[][])  [unwired: 1 in, 1 out]
                  n175 = Insert Into Array(array=w427, new element=w425) -> (w426:string[][])  [unwired: 2 in]
                  n176 = in-place-cluster #7("Formular"=w426) -> (w422:T7)
                }
              }
            }
          }
          frame Error {
          }
        }
      }
      frame "Formular Delete" {
        n177 = in-place {
          in-place-border: w434 -> [w444]
          in-place-border: ["Formular Save"] -> w433
          n178 = in-place-cluster #8(w434) -> ("Formular"=w445:string[][])
          n179 = Unbundle By Name(w444) -> ("FormularRef"=w443:refnum<vi>)
          n180 = property class="MCListbox"(reference=w443) -> ("Value"=w442:variant)  [unwired: 1 in, 2 out]
          n181 = Variant To Data(type=0, Variant=w442) -> (data=w440:i32)  [unwired: 1 in, 1 out]
          n182 = Delete From Array(array=w445, index (row)=w440) -> (array with subset deleted=w439:string[][])  [unwired: 2 in, 1 out]
          n183 = in-place-cluster #8("Formular"=w439) -> (w435:T7)
        }
      }
      frame "Panel Change" {
        n184 = call "MCList Adjust.vi"() -> ()  [unwired: 11 in, 1 out]
      }
      frame "Exit" {
        n185 = Unbundle By Name(w449) -> ("Queue.Message"=w454:refnum<queue>, "Queue.Data"=w453:refnum<queue>)
        n186 = Build Array(w454, w453) -> (w452:refnum<queue>[])
        n187 = Unbundle By Name(w449) -> ("Queue.UE"=w450:refnum<user-event>)
        n188 = for {
          tunnel: w452 -> [w461] mode=indexing
          tunnel: w451 -> [w460]
          n189 = call "Queue In.vi"("Message"=w460, "Queue In"=w461) -> ()  [unwired: 8 in, 2 out]
        }
        n190 = Generate User Event(user event=w450, event data cluster=w451) -> ()  [unwired: 2 in, 2 out]
        n191 = call "Queue Clear.vi"("error in (no error)"=w456, "Queue In"=w458) -> ("error out"=w455:errorcluster, "Queue Out"=w457:refnum<queue>)  [unwired: 8 in]
      }
      frame "Quit" {
      }
    }
    n192 = call "Queue In.vi"("error in (no error)"=w195, "Data"=w193, "Message"=w194, "Queue In"=w198) -> ("error out"=w196:errorcluster, "Queue Out"=w197:refnum<queue>)  [unwired: 6 in]
  }
  n193 = call "000 Driver Message.vi"("Queue In"=w1) -> ("error out"=w19:errorcluster)  [unwired: 8 in, 2 out]
  n194 = call "Queue Release.vi"("error in (no error)"=w16, "Queue In"=w15) -> ("error out"=w18:errorcluster)  [unwired: 9 in]
  n195 = call "Queue Release.vi"("error in (no error)"=w8, "Queue In"=w7) -> ("error out"=w11:errorcluster)  [unwired: 9 in]
  n196 = Unregister For Events(event registration refnum=w5) -> (error out=w6:errorcluster)  [unwired: 1 in]
  n197 = Destroy User Event(user event=w2, error in=w6) -> (error out=w10:errorcluster)
  n198 = Call Chain() -> (call chain=w13:string[])
  n199 = Merge Errors(w10, w11, w19, w18) -> (w12:errorcluster)
  n200 = Array Size(array=w13) -> (size(s)=w14:i32)
  n201 = case shown="2.." w14 {
    tunnel: w12 -> [_ w466]
    frame 0, Default {
    }
    frame 2.. {
      n202 = invoke class="VI" method="FP.Close"(error in=w466) -> ()  [unwired: 2 in, 3 out]
    }
  }
